vi "Get Data Variant.vi"(8 "error in (no error)":errorcluster, 11 "UDP Thread Configuration in":refnum<class "UDP Thread Configuration.lvclass">) -> (0 "error out":errorcluster, 1 "data version":T1, 2 "data":variant, 3 "UDP Thread Configuration out":refnum<class "UDP Thread Configuration.lvclass">)   [LabVIEW 2017, in "UDP Transceiver.lvlib" / "UDP Thread Configuration.lvclass"]
uses:
  UDP Thread Configuration.lvclass
  DSF Core.lvlibp/Typedefs/DSF Version Info.ctl
  DSF Core.lvlibp/Classes/Configuration/Configuration.lvclass
  DSF Core.lvlibp
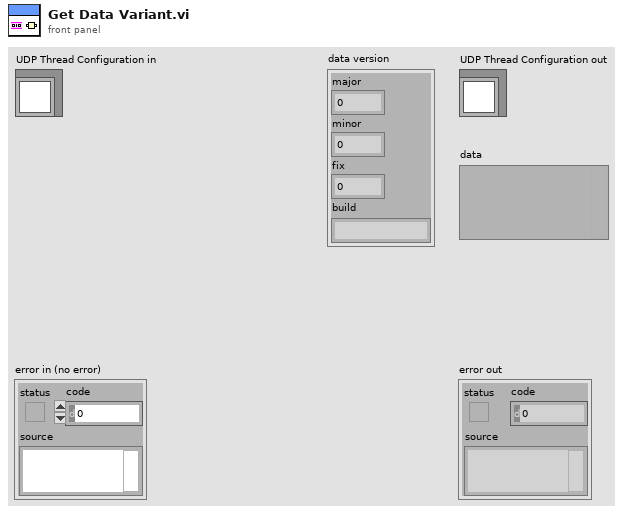
[diagram p1: front panel]
types:
  T1 = typedef "DSF Core.lvlibp/DSF Version Info.ctl" = cluster{"major":u32, "minor":u32, "fix":u32, "build":string}
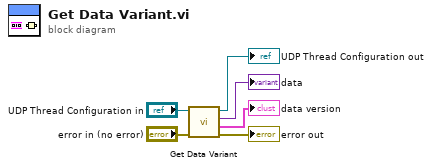
[diagram p0: block diagram]
diagram:
  n1 = call-parent "Get Data Variant.vi"("error in (no error)"="error in (no error)", "Configuration in"="UDP Thread Configuration in") -> ("error out"=→"error out":errorcluster, "data version"=→"data version":T1, "data"=→"data":variant, "Configuration out"=→"UDP Thread Configuration out":refnum<class "UDP Thread Configuration.lvclass">)  [unwired: 6 in]
